vi "from_json.vi"(8 "error in":errorcluster, 10 "json":string, 11 "labels in":refnum<class "labels.lvclass">) -> (0 "error out":errorcluster, 3 "labels out":refnum<class "labels.lvclass">)   [LabVIEW 2020, in "nominal types.lvlib" / "labels.lvclass"]
uses:
  labels.lvclass
  1dbc0355-b049-4ca1-933e-7ee337e7c81e.vi
  <vilib>/JDP Science/JSONtext/JSON text to Variant.vi
  <vilib>/JDP Science/JSONtext/LVClass Serializer/JSONtext LVClass Serializer.lvclass
  labels.lvclass/labels.ctl
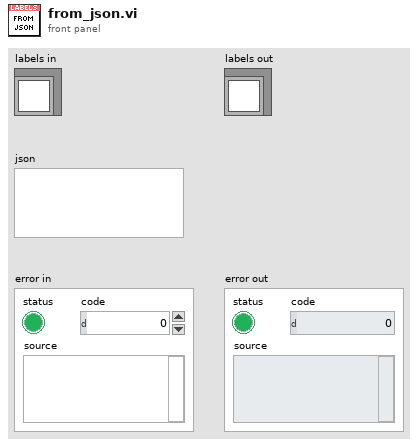
[diagram p1: front panel]
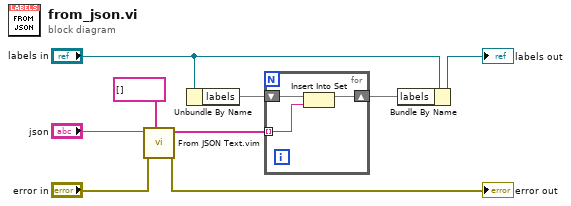
[diagram p0: block diagram]
diagram:
  n1 = call "From JSON Text.vim"("Data Type and Default Value"=string[] [], "error in (no error)"="error in", "JSON"="json") -> ("error out"=→"error out":errorcluster, "Data out"=w6:string[])  [unwired: 7 in]
  n2 = Unbundle By Name("labels in") -> ("labels"=w7:set{string})
  n3 = for {
    shift-right: [w10] -> w4
    shift-left: w7 -> [w12]
    tunnel: w6 -> [w11] mode=indexing
    n4 = Insert Into Set(10:w11, 11:w12) -> (3:w10:set{string})  [unwired: 1 out]
  }
  n5 = Bundle By Name(cluster="labels in", "labels"=w4) -> (→"labels out":refnum<class "labels.lvclass">)
